vi "Main.vi"(11 "Module Admin":refnum<class "Delacor_lib_QMH_Module Admin.lvclass">) -> ()   [LabVIEW 2018, in "Storage.lvlib"]
doc: "This template is based off of the Queued Message Handler design pattern and the Queued Message Handler project template that ships with LabVIEW.\n\nThe main difference is that the queue is private to this module and communication between modules is performed via Broadcast and Request events.\n\nRequest events are wrapped in public API methods and are handled in the Event Handling Loop (EHL) of this VI. Any module can register for Broadcast events sent by this module. The EHL generates messages based on user interface actions.\n\nThe Message Handling Loop (MHL) processes messages generated by the EHL, or by other messages. The messages are string values, so new messages can be added easily to the Message Cases case structure in the MHL. Each message cluster can also provide an optional value for Message Data, which is a variant that can be converted to whatever message-specific data is required.\n_____\nBased on DQMH Project Template 6.1.0.94."
uses:
  Storage.lvlib
  <vilib>/Delacor/Delacor QMH/Libraries/Module Admin_class/Delacor_lib_QMH_Module Admin.lvclass
  Module Data--cluster.ctl
  <vilib>/drjdpowell/SQLite Library/SQL Connection/Connection.lvclass
  <vilib>/Delacor/Delacor QMH/Libraries/Message Queue_class/Delacor_lib_QMH_Message Queue.lvclass/Delacor_lib_QMH_Message Queue.ctl
  Stop Argument--cluster.ctl
  <vilib>/Delacor/Delacor QMH/Libraries/Module Admin_class/Delacor_lib_QMH_Module Admin.lvclass/Delacor_lib_QMH_Module Admin.ctl
  Get TDMS Ref Argument--cluster.ctl
  Get TDMS Ref (Reply Payload)--cluster.ctl
  <vilib>/Utility/miscctls.llb/LVPointTypeDef.ctl
  <vilib>/Utility/sysdir.llb/System Directory Type.ctl
  <vilib>/Delacor/Delacor QMH/Libraries/Message Queue_class/Delacor_lib_QMH_Enqueue Message (Single).vi
  <vilib>/Delacor/Delacor QMH/Libraries/Module Admin_class/Delacor_lib_QMH_Get External Launch.vi
  <vilib>/Delacor/Delacor QMH/Libraries/Message Queue_class/Delacor_lib_QMH_Enqueue Message (Array).vi
  <vilib>/Utility/error.llb/Error Cluster From Error Code.vi
  <vilib>/ErrorRing/Error Ring.xnode
  <vilib>/Delacor/Delacor QMH/Libraries/Message Queue_class/Delacor_lib_QMH_Message Queue.lvclass
panel:
  out "error out":errorcluster
  out "Status":string
  in  "Simulate MHL Error":bool
  in  "Simulate EHL Error":bool
  # "Other QMH Modules communicate with this Module via its Public API (wrappers for its Request Events).\n\nThis Module communicates with other Modules via its Broadcast Events.\nAny module that wants to get these messages, just registers for this module's Broadcast events."
  # "This template is for the Delacor Modified Queued Message Handler design pattern.\n\nSee the block diagram for more information on how to use this template."
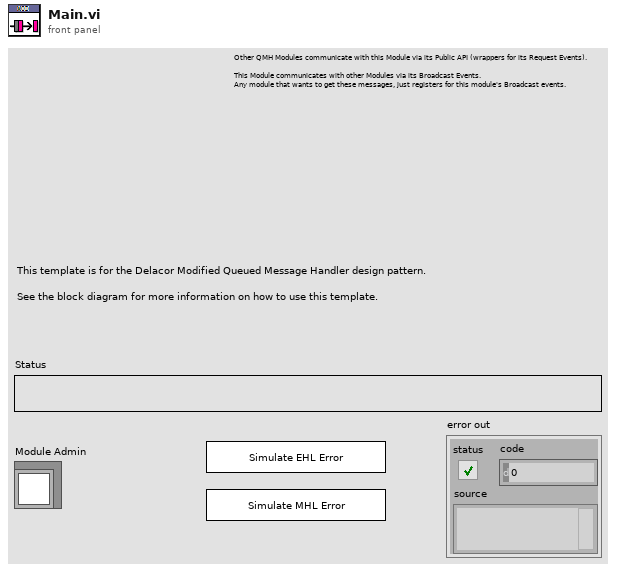
[diagram p1: front panel]
types:
  T1 = typedef "Storage.lvlib/Module Data--cluster.ctl" = cluster{"Status":string, "Data Path":path, "TDMS原":refnum<k34>[], "TDMS实":refnum<k34>[], "DB Con":refnum<class "Connection.lvclass">}
  T2 = typedef "Storage.lvlib/Request Events--cluster.ctl" = cluster{"Stop Module":refnum<user-event>, "Show Panel":refnum<user-event>, "Hide Panel":refnum<user-event>, "Get Module Execution Status":refnum<user-event>, "Show Diagram":refnum<user-event>, "Wakeup or Sleep HL":refnum<user-event>, "Get TDMS Ref":refnum<user-event>}
  T3 = enum32{"invalid lock state", "Not Locked", "Locked (No Password)", "Password-protected"}
  T4 = typedef "Storage.lvlib/Stop Argument--cluster.ctl" = cluster{"Origin":string, "Exit via Stop Module Req?":bool, "Wait for Module to stop?":bool}
  T5 = typedef "Storage.lvlib/Get TDMS Ref Argument--cluster.ctl" = cluster{"TDMS ID":i32, "Wait Notifier":refnum<notifier>, "wait for reply":bool}
  T6 = typedef "LVPointTypeDef.ctl" = cluster{"Horizontal":i16, "Vertical":i16}
  T7 = enum32{"Invalid", "Standard", "Closed", "Hidden", "Minimized", "Maximized"}
  T8 = enum16{"open", "open or create", "create or replace", "create", "open (read-only)"}
  T9 = typedef "Storage.lvlib/Get TDMS Ref (Reply Payload)--cluster.ctl" = cluster{"TDMS":refnum<k34>, "error":errorcluster}
  T10 = typedef "System Directory Type.ctl" = i32
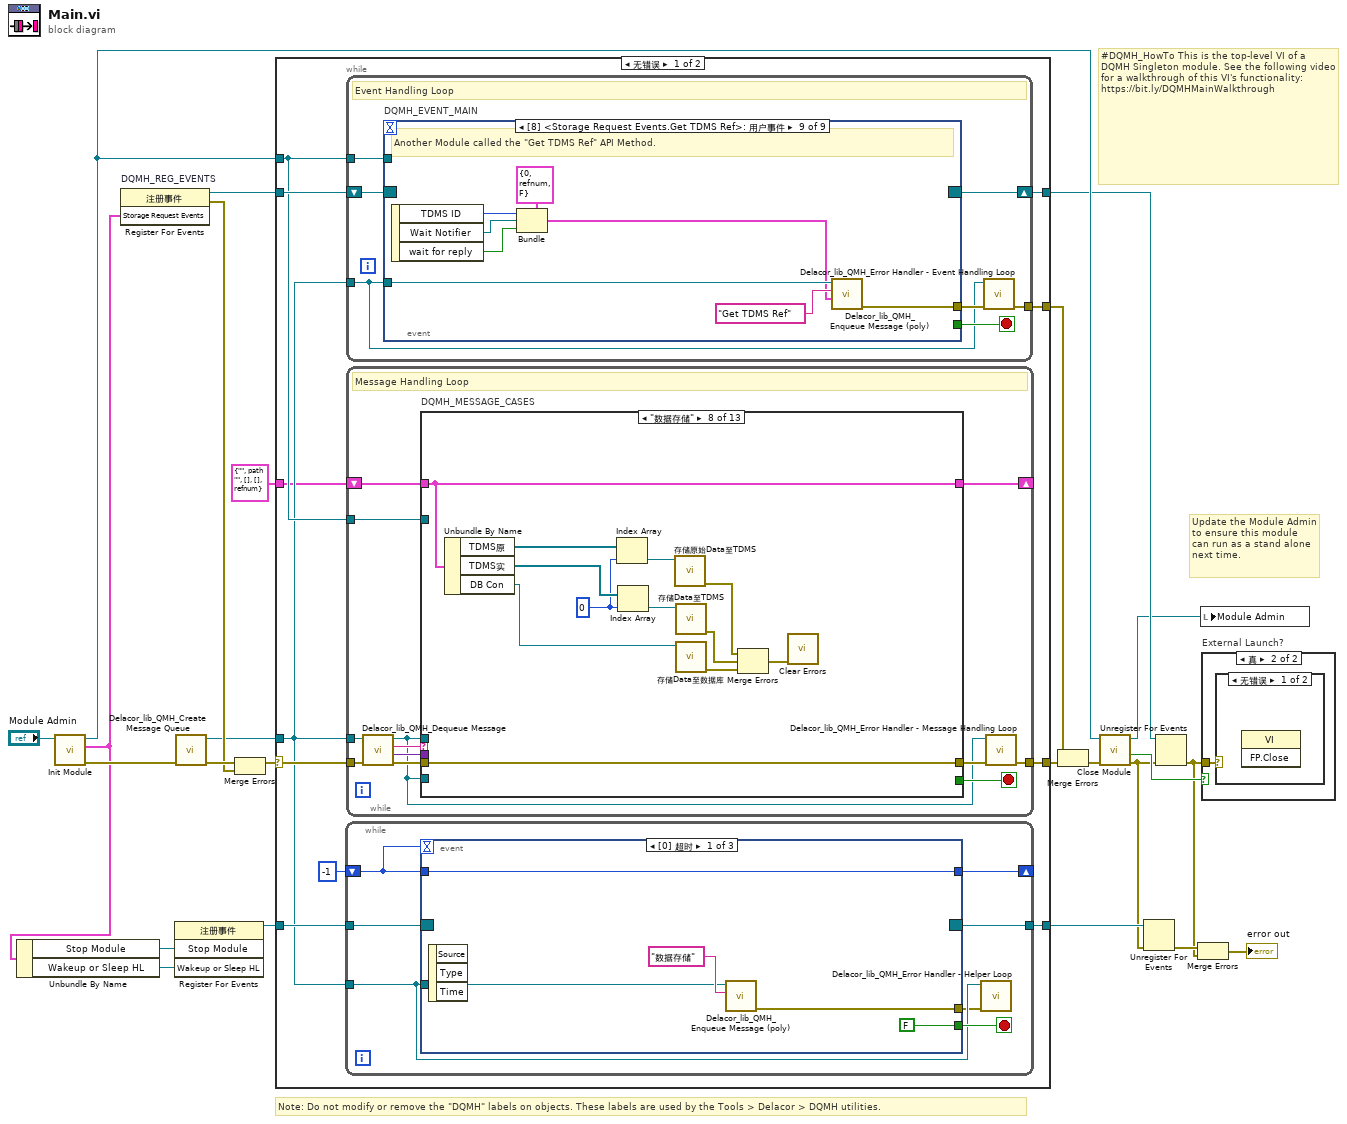
[diagram p0: block diagram]
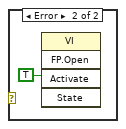
[diagram p3: hidden frame]
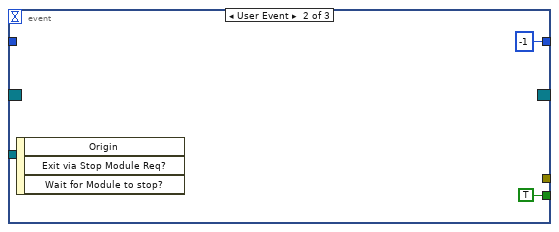
[diagram p4: hidden frame]
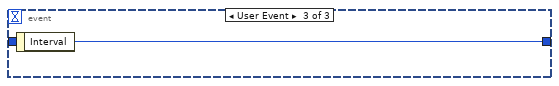
[diagram p5: hidden frame]
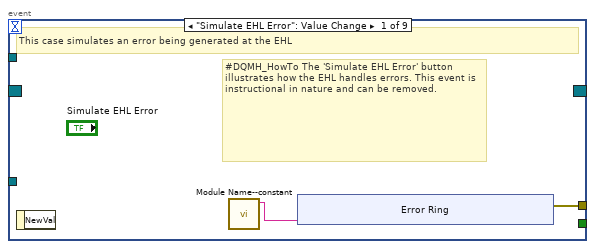
[diagram p6: hidden frame]
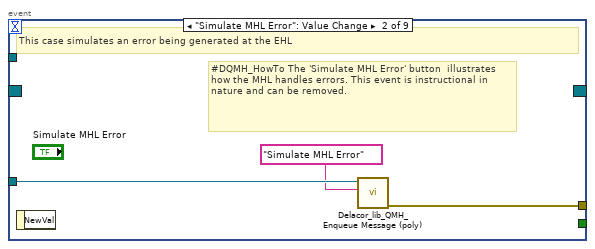
[diagram p7: hidden frame]
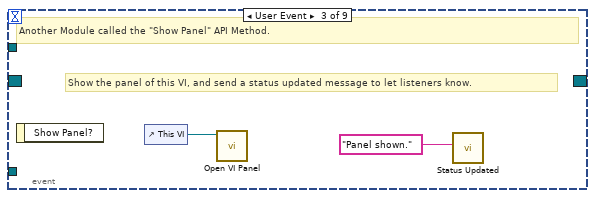
[diagram p8: hidden frame]
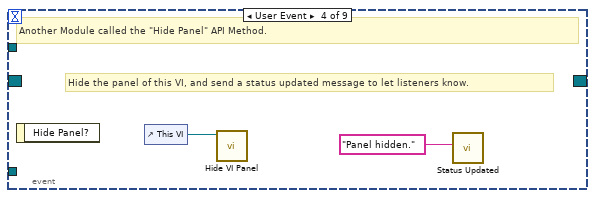
[diagram p9: hidden frame]
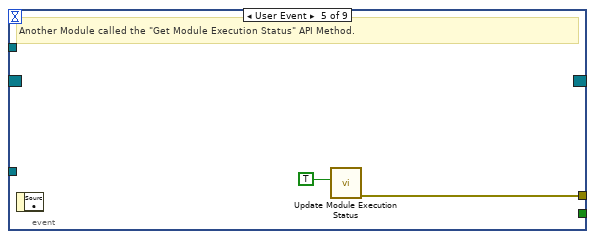
[diagram p10: hidden frame]
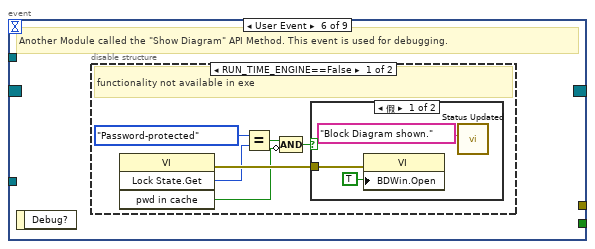
[diagram p11: hidden frame]
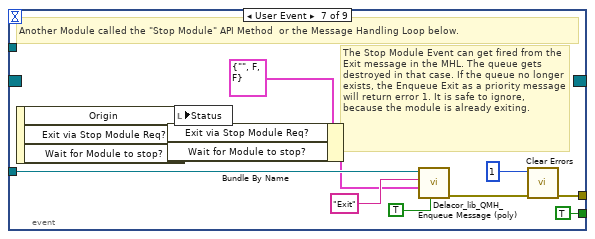
[diagram p14: hidden frame]
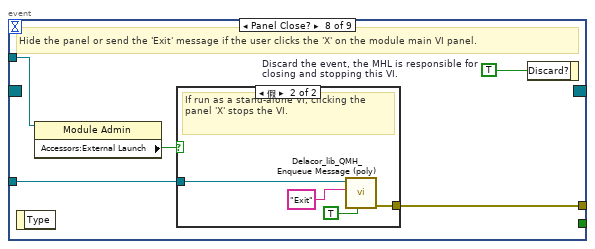
[diagram p15: hidden frame]
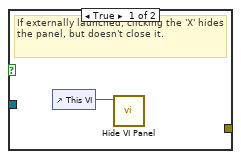
[diagram p16: hidden frame]
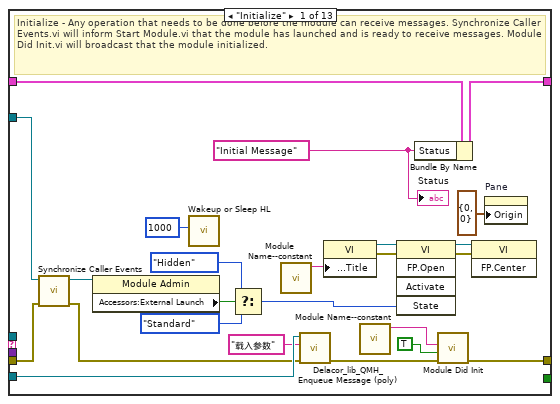
[diagram p17: hidden frame]
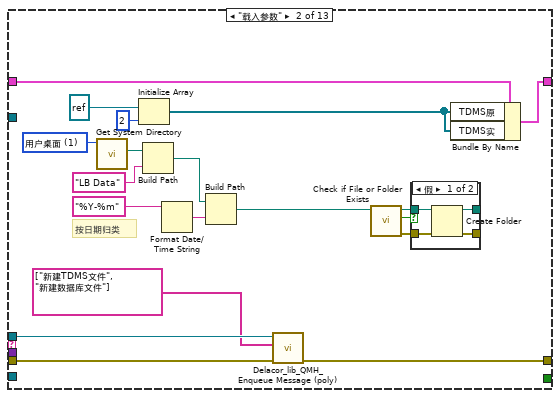
[diagram p18: hidden frame]
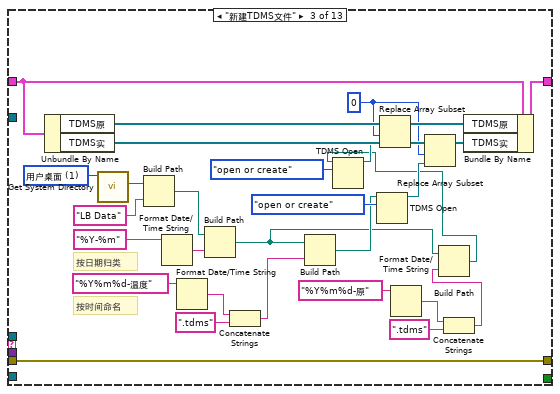
[diagram p20: hidden frame]
diagram:
  # "#DQMH_HowTo This is the top-level VI of a DQMH Singleton module. See the following video for a walkthrough of this VI's functionality: https://bit.ly/DQMHMainWalkthrough"
  # "Note: Do not modify or remove the \"DQMH\" labels on objects. These labels are used by the Tools > Delacor > DQMH utilities."
  # "Update the Module Admin to ensure this module can run as a stand alone next time."
  n1 = call "Init Module.vi"("Singleton Module Admin in"="Module Admin") -> ("error out"=w23:errorcluster, "Storage Request Events"=w7:T2, "Singleton Module Admin out"=w17:refnum<class "Delacor_lib_QMH_Module Admin.lvclass">)  [unwired: 8 in]
  n2 = Unbundle By Name ("按名称解除捆绑")(w7) -> ("Stop Module"=w10:refnum<user-event>, "Wakeup or Sleep HL"=w9:refnum<user-event>)
  n3 = register-events "DQMH_REG_EVENTS"(w7) -> (reference out=w15:refnum<event-registration>, error out=w18:errorcluster)  [unwired: 2 in]
  n4 = register-events ("注册事件")(w10, w9) -> (reference out=w8:refnum<event-registration>)  [unwired: 2 in, 1 out]
  n5 = call <vilib>:"Delacor_lib_QMH_Create Message Queue.vi"("error in"=w23) -> ("error out"=w20:errorcluster, "Message Queue"=w14:refnum<class "Delacor_lib_QMH_Message Queue.lvclass">)  [unwired: 9 in]
  n6 = Merge Errors(w20, w18) -> (w19:errorcluster)
  n7 = case shown="无错误" w19 {
    selector: w19 -> [w33 w313]
    tunnel: [w35 w312] -> w24
    tunnel: [w32 w318] -> w16
    tunnel: w15 -> [w31 w318]
    tunnel: w14 -> [w27 w311]
    tunnel: [w34 _] -> w22
    tunnel: w17 -> [w30 w314]
    tunnel: w8 -> [w28 w310]
    tunnel: [w26 w310] -> w5
    tunnel: T1 {"Status"="", "Data Path"=path "", "TDMS原"=[], "TDMS实"=[], "DB Con"=refnum} ("Data Cluster") -> [w25 _]
    frame No Error {
      n8 = while {
        shift-right: [w41] -> _
        shift-left: -1 ("Interval") -> [w42]
        tunnel: w28 -> [w39]
        tunnel: [w38] -> w26
        tunnel: w27 -> [w37]
        stop <- w40 stop-if-true
        n9 = event "事件结构" shown="[0] 超时" {
          selector: w39 -> [_ _ _]
          dyn-events: [_ _ _] -> w38
          timeout: w42 -> [_ _ _]
          tunnel: w42 -> [w43 _ _]
          tunnel: [w43 -1 w50] -> w41
          tunnel: [FALSE TRUE _] -> w40
          tunnel: w37 -> [w45 _ _]
          tunnel: [w44 _ _] -> w36
          event Timeout {
            n10 = event-data() -> ()  [unwired: 1 in, 3 out]
            n11 = call-poly <vilib>:"Delacor_lib_QMH_Enqueue Message (poly).vi"("Message"="数据存储", "Message Queue in"=w45) -> ("error out"=w44:errorcluster)  [unwired: 8 in, 1 out]
          }
          event User Event {
            n12 = event-data() -> ()  [unwired: 1 in, 3 out]
          }
          event User Event {
            n13 = event-data() -> ("Interval"=w50:i32)  [unwired: 1 in]
          }
        }
        n14 = call-dynamic "Delacor_lib_QMH_Error Handler - Helper Loop.vi"("error in"=w36, "Message Queue in"=w37) -> ()  [unwired: 8 in, 2 out]
      }
      n15 = while {
        tunnel: w27 -> [w51]
        shift-right: [w54] -> w32
        shift-left: w31 -> [w55]
        tunnel: [w56] -> w34
        tunnel: w30 -> [w52]
        stop <- w53 stop-if-true
        # "Event Handling Loop"
        n16 = event "DQMH_EVENT_MAIN" shown="[8] <Storage Request Events.Get TDMS Ref>: 用户事件" {
          selector: w55 -> [_ _ _ _ _ _ _ _ _]
          dyn-events: [_ _ _ _ _ _ _ _ _] -> w54
          timeout: _ -> [_ _ _ _ _ _ _ _ _]
          tunnel: [_ _ _ _ _ _ TRUE ("Discard?") _ _] -> w53
          tunnel: w51 -> [_ w68 _ _ _ _ w92 w99 w114]
          tunnel: [w59 w69 _ _ w75 _ w95 w101 w107] -> w57
          tunnel: w52 -> [_ _ _ _ _ _ _ w98 _]
          event "Simulate EHL Error": Value Change {
            # "#DQMH_HowTo The 'Simulate EHL Error' button  illustrates how the EHL handles errors. This event is instructional in nature and can be removed."
            # "This case simulates an error being generated at the EHL"
            n17 = event-data() -> ()  [unwired: 1 in, 1 out]
            n18 = call "Module Name--constant.vi"() -> ("Module Name"=w58:string)  [unwired: 11 in]
            n19 = xnode "Error Ring"("参数 0"=w58) -> ("错误输出"=w59:errorcluster)
          }
          event "Simulate MHL Error": Value Change {
            # "#DQMH_HowTo The 'Simulate MHL Error' button  illustrates how the MHL handles errors. This event is instructional in nature and can be removed."
            # "This case simulates an error being generated at the EHL"
            n20 = event-data() -> ()  [unwired: 1 in, 1 out]
            n21 = call-poly <vilib>:"Delacor_lib_QMH_Enqueue Message (poly).vi"("Message"="Simulate MHL Error", "Message Queue in"=w68) -> ("error out"=w69:errorcluster)  [unwired: 8 in, 1 out]
          }
          event User Event {
            # "Show the panel of this VI, and send a status updated message to let listeners know."
            # "Another Module called the \"Show Panel\" API Method."
            n22 = event-data() -> ()  [unwired: 1 in, 1 out]
            n23 = control-ref of="This VI"() -> (w71:refnum<vi>)
            n24 = call "Open VI Panel.vi"("VI"=w71) -> ()  [unwired: 10 in, 1 out]
            n25 = call "Status Updated.vi"("Status"="Panel shown." ("format string")) -> ()  [unwired: 10 in, 1 out]
          }
          event User Event {
            # "Hide the panel of this VI, and send a status updated message to let listeners know."
            # "Another Module called the \"Hide Panel\" API Method."
            n26 = event-data() -> ()  [unwired: 1 in, 1 out]
            n27 = control-ref of="This VI"() -> (w73:refnum<vi>)
            n28 = call "Hide VI Panel.vi"("VI"=w73) -> ()  [unwired: 10 in, 1 out]
            n29 = call "Status Updated.vi"("Status"="Panel hidden." ("format string")) -> ()  [unwired: 10 in, 1 out]
          }
          event User Event {
            # "Another Module called the \"Get Module Execution Status\" API Method."
            n30 = event-data() -> ()  [unwired: 1 in, 1 out]
            n31 = call "Update Module Execution Status.vi"("Running?"=TRUE) -> ("error out"=w75:errorcluster)  [unwired: 10 in]
          }
          event User Event {
            # "Another Module called the \"Show Diagram\" API Method. This event is used for debugging."
            n32 = event-data() -> ()  [unwired: 1 in, 1 out]
            n33 = disable-structure shown="RUN_TIME_ENGINE==False" {
              frame condition #0 (active) {
                # "functionality not available in exe"
                n34 = invoke class="VI" method="Lock State.Get"() -> (error out=w81:errorcluster, "Get Lock State"=w80:T3, "pwd in cache"=w77:bool)  [unwired: 4 in, 1 out]
                n35 = Equal?(x=T3."Password-protected", y=w80) -> (x = y?=w78:bool)
                n36 = Compound Arithmetic op=AND(w78, invert w77) -> (w76:bool)
                n37 = case "条件结构" shown="假" w76 {
                  tunnel: w81 -> [w84 _]
                  frame False {
                    n38 = property class="VI"(error in=w84, "BDWin.Open"=TRUE ("Block Diagram Window:Open")) -> ()  [unwired: 1 in, 2 out]
                    n39 = call "Status Updated.vi"("Status"="Block Diagram shown." ("format string")) -> ()  [unwired: 10 in, 1 out]
                  }
                  frame True {
                    # "Password-protected VI, and the password is not in the cache. Do not show the diagram."
                  }
                }
              }
              frame condition #1 {
              }
            }
          }
          event User Event {
            # "The Stop Module Event can get fired from the Exit message in the MHL. The queue gets destroyed in that case. If the queue no longer exists, the Enqueue Exit as a priority message will return error 1. It is safe to ignore, because the module is already exiting."
            # "Another Module called the \"Stop Module\" API Method  or the Message Handling Loop below."
            n40 = event-data() -> ("Origin"=w91:string, "Exit via Stop Module Req?"=w87:bool, "Wait for Module to stop?"=w86:bool)  [unwired: 1 in]
            n41 = Bundle By Name(cluster=T4 {"Origin"="", "Exit via Stop Module Req?"=FALSE, "Wait for Module to stop?"=FALSE} ("Stop Argument"), "Exit via Stop Module Req?"=w87, "Wait for Module to stop?"=w86) -> (w85:T4)
            n42 = local write "Status"(w91) -> ()
            n43 = call-poly <vilib>:"Delacor_lib_QMH_Enqueue Message (poly).vi"("Priority Message? (F)"=TRUE, "Message Data"=w85, "Message"="Exit", "Message Queue in"=w92) -> ("error out"=w96:errorcluster)  [unwired: 6 in, 1 out]
            n44 = call <vilib>:"Clear Errors.vi"("error in (no error)"=w96, "specific error code to clear (0: all)"=1) -> ("error out"=w95:errorcluster)  [unwired: 4 in, 1 out]
          }
          event Panel Close? {
            w100 = TRUE  # Discard the event, the MHL is responsible for closing and stopping this VI.
            # "Hide the panel or send the 'Exit' message if the user clicks the 'X' on the module main VI panel."
            n45 = event-data() -> ()  [unwired: 1 in, 1 out]
            n46 = property class="Module Admin"(reference=w98) -> ("Accessors:External Launch"=w97:bool)  [unwired: 1 in, 2 out]
            n47 = case "条件结构" shown="假" w97 {
              tunnel: w99 -> [_ w105]
              tunnel: [_ w106] -> w101
              frame True {
                # "If externally launched, clicking the 'X' hides the panel, but doesn't close it."
                n48 = control-ref of="This VI"() -> (w102:refnum<vi>)
                n49 = call "Hide VI Panel.vi"("VI"=w102) -> ()  [unwired: 10 in, 1 out]
              }
              frame False {
                # "If run as a stand-alone VI, clicking the panel 'X' stops the VI."
                n50 = call-poly <vilib>:"Delacor_lib_QMH_Enqueue Message (poly).vi"("Priority Message? (F)"=TRUE, "Message"="Exit", "Message Queue in"=w105) -> ("error out"=w106:errorcluster)  [unwired: 7 in, 1 out]
              }
            }
            n51 = event-data("Discard?"=w100) -> ()  [unwired: 1 in, 1 out]
          }
          event User Event {
            # "Another Module called the \"Get TDMS Ref\" API Method."
            n52 = event-data() -> ("TDMS ID"=w110:i32, "Wait Notifier"=w109:refnum<notifier>, "wait for reply"=w108:bool)  [unwired: 1 in]
            n53 = Bundle(cluster=T5 {"TDMS ID"=0, "Wait Notifier"=refnum, "wait for reply"=FALSE} ("Get TDMS Ref Argument"), "TDMS ID"=w110, "Wait Notifier"=w109, "wait for reply"=w108) -> (w111:T5)
            n54 = call-poly <vilib>:"Delacor_lib_QMH_Enqueue Message (poly).vi"("Message Data"=w111, "Message"="Get TDMS Ref", "Message Queue in"=w114) -> ("error out"=w107:errorcluster)  [unwired: 7 in, 1 out]
          }
        }
        n55 = call-dynamic "Delacor_lib_QMH_Error Handler - Event Handling Loop.vi"("error in"=w57, "Message Queue in"=w51) -> ("dup error in"=w56:errorcluster)  [unwired: 8 in, 1 out]
      }
      n56 = while {
        tunnel: w27 -> [w117]
        shift-right: [w121] -> _
        shift-left: w25 -> [w122]
        tunnel: w33 -> [w125]
        tunnel: [w123] -> w35
        tunnel: w30 -> [w116]
        stop <- w120 stop-if-true
        # "Message Handling Loop"
        n57 = call-dynamic "Delacor_lib_QMH_Dequeue Message.vi"("error in"=w125, "Message Queue in"=w117) -> ("error out"=w124:errorcluster, "Message Data"=w118:variant, "Message"=w119:string, "Message Queue out"=w115:refnum<class "Delacor_lib_QMH_Message Queue.lvclass">)  [unwired: 6 in]
        n58 = case "DQMH_MESSAGE_CASES" shown="\"数据存储\"" w119 {
          selector: w119 -> [_ _ _ _ _ _ _ _ _ _ _ _ w297]
          tunnel: w115 -> [_ w159 _ _ _ _ _ _ _ _ w258 w283 _]
          tunnel: w124 -> [w148 w158 w204 w208 w210 w224 w229 w239 w243 w248 w265 w289 w299]
          tunnel: [w147 w157 w204 w208 w210 w215 w228 w239 w243 w247 w261 w286 w300] -> w126
          tunnel: w122 -> [w138 w167 w189 w207 w209 w214 w227 w241 w242 w245 w260 w275 w298]
          tunnel: [w137 w166 w191 w206 w209 w214 w227 w241 w242 w245 w260 w275 w298] -> w121
          tunnel: [_ _ _ _ _ _ _ _ _ _ _ w282 _] -> w120
          tunnel: w118 -> [_ _ _ _ _ w222 _ _ _ _ w259 w281 _]
          tunnel: w116 -> [w139 _ _ _ _ _ _ _ _ _ w257 w276 _]
          tunnel: w115 -> [w130 _ _ _ _ _ _ _ _ _ _ _ _]
          frame "Initialize" {
            w133 = "Initial Message" ("Initial Message")
            # "Initialize - Any operation that needs to be done before the module can receive messages. Synchronize Caller Events.vi will inform Start Module.vi that the module has launched and is ready to receive messages. Module Did Init.vi will broadcast that the module initialized."
            n59 = call "Synchronize Caller Events.vi"("error in (no error)"=w148, "Singleton Module Admin in"=w139) -> ("error out"=w129:errorcluster, "Singleton Module Admin out"=w134:refnum<class "Delacor_lib_QMH_Module Admin.lvclass">)  [unwired: 8 in]
            n60 = property class="Module Admin"(reference=w134) -> ("Accessors:External Launch"=w143:bool)  [unwired: 1 in, 2 out]
            n61 = call "Wakeup or Sleep HL.vi"("Interval"=1000) -> ()  [unwired: 10 in, 1 out]
            n62 = Select(t=T7."Hidden" ("State"), s=w143, f=T7."Standard" ("State")) -> (s? t:f=w140:T7)
            n63 = call "Module Name--constant.vi"() -> ("Module Name"=w146:string)  [unwired: 11 in]
            n64 = call-poly <vilib>:"Delacor_lib_QMH_Enqueue Message (poly).vi"("error in"=w129, "Message"="载入参数", "Message Queue in"=w130) -> ("error out"=w128:errorcluster)  [unwired: 7 in, 1 out]
            n65 = property class="VI"("Front Panel.Title"=w146) -> (reference out=w145:refnum<vi>, error out=w150:errorcluster)  [unwired: 2 in]
            n66 = call "Module Name--constant.vi"() -> ("Module Name"=w135:string)  [unwired: 11 in]
            n67 = invoke class="VI" method="FP.Open"(reference=w145, error in=w150, "State"=w140) -> (reference out=w144:refnum<vi>, error out=w149:errorcluster)  [unwired: 2 in, 3 out]
            n68 = Bundle By Name(cluster=w138, "Status"=w133) -> (w137:T1)
            n69 = call "Module Did Init.vi"("error in (no error)"=w128, "Initialized?"=TRUE, "Origin"=w135) -> ("error out"=w147:errorcluster)  [unwired: 8 in]
            n70 = invoke class="VI" method="FP.Center"(reference=w144, error in=w149) -> ()  [unwired: 1 in, 3 out]
            n71 = property on="Pane" class="Pane"("Origin"=T6 {"Horizontal"=0, "Vertical"=0}) -> ()  [unwired: 2 in, 2 out]
            "Status" <- w133
          }
          frame "载入参数" {
            w165 = T10 1 items=["用户目录"=0, "用户桌面"=1, "用户文档"=2, "用户应用程序数据"=3, "用户设置"=4, "用户临时目录"=5, "公共文档"=6, "公共应用程序数据"=7, "公共设置"=8, "公共缓存"=13, "系统核心库"=9, "系统安装库"=10, "应用程序文件"=11, "启动盘根目录"=12] ("system directory type")
            # "按日期归类"
            n72 = call <vilib>:"Get System Directory.vi"("system directory type"=w165) -> ("system directory"=w164:path)  [unwired: 10 in]
            n73 = Initialize Array(refnum<k34> refnum ("TDMS"), 2 ("维数大小")) -> (w151:refnum<k34>[])
            n74 = Build Path(base path=w164, name or relative path="LB Data" ("名称或相对路径")) -> (appended path=w160:path)
            n75 = Format Date/Time String(time format string (%c)="%Y-%m" ("时间格式字符串(%c)")) -> (date/time string=w161:string)  [unwired: 2 in]
            n76 = Build Path(base path=w160, name or relative path=w161) -> (appended path=w152:path)
            n77 = call-poly <vilib>:"Delacor_lib_QMH_Enqueue Message (poly).vi"("error in"=w158, "Message Array"=string[] ["新建TDMS文件", "新建数据库文件"] ("Message"), "Message Queue in"=w159) -> ("error out"=w157:errorcluster)  [unwired: 7 in, 1 out]
            n78 = call <vilib>:"Check if File or Folder Exists.vi"("path"=w152) -> ("error out"=w154:errorcluster, "file or folder exists?"=w155:bool, "dup path"=w153:path)  [unwired: 8 in]
            n79 = case shown="假" w155 {
              tunnel: w153 -> [w173 w174]
              tunnel: w154 -> [w172 w175]
              tunnel: [w171 w175] -> _
              tunnel: [w170 w174] -> _
              frame False {
                n80 = Create Folder(path (use dialog)=w173, error in=w172) -> (created path=w170:path, error out=w171:errorcluster)  [unwired: 1 in, 1 out]
              }
              frame True {
              }
            }
            n81 = Bundle By Name(cluster=w167, "TDMS原"=w151, "TDMS实"=w151) -> (w166:T1)
          }
          frame "新建TDMS文件" {
            w184 = 0 ("索引")
            w203 = T10 1 items=["用户目录"=0, "用户桌面"=1, "用户文档"=2, "用户应用程序数据"=3, "用户设置"=4, "用户临时目录"=5, "公共文档"=6, "公共应用程序数据"=7, "公共设置"=8, "公共缓存"=13, "系统核心库"=9, "系统安装库"=10, "应用程序文件"=11, "启动盘根目录"=12] ("system directory type")
            # "按时间命名"
            # "按日期归类"
            n82 = Unbundle By Name(w189) -> ("TDMS原"=w186:refnum<k34>[], "TDMS实"=w188:refnum<k34>[])
            n83 = call <vilib>:"Get System Directory.vi"("system directory type"=w203) -> ("system directory"=w202:path)  [unwired: 10 in]
            n84 = Build Path(base path=w202, name or relative path="LB Data" ("名称或相对路径")) -> (appended path=w198:path)
            n85 = Format Date/Time String(time format string (%c)="%Y-%m" ("时间格式字符串(%c)")) -> (date/time string=w199:string)  [unwired: 2 in]
            n86 = Format Date/Time String(time format string (%c)="%Y%m%d-温度" ("时间格式字符串(%c)")) -> (date/time string=w196:string)  [unwired: 2 in]
            n87 = Build Path(base path=w198, name or relative path=w199) -> (appended path=w178:path)
            n88 = Concatenate Strings(w196, ".tdms" ("字符串")) -> (w194:string)
            n89 = Build Path(base path=w178, name or relative path=w194) -> (appended path=w192:path)
            n90 = TDMS Open(10:T8."open or create" ("操作(0:open)"), 11:w192) -> (3:w187:refnum<k34>)  [unwired: 5 in, 1 out]
            n91 = Format Date/Time String(time format string (%c)="%Y%m%d-原" ("时间格式字符串(%c)")) -> (date/time string=w180:string)  [unwired: 2 in]
            n92 = Replace Array Subset(array=w188, new element=w187, index=w184) -> (w190:refnum<k34>[])
            n93 = Concatenate Strings(w180, ".tdms" ("字符串")) -> (w177:string)
            n94 = Build Path(base path=w178, name or relative path=w177) -> (appended path=w176:path)
            n95 = TDMS Open(10:T8."open or create" ("操作(0:open)"), 11:w176) -> (3:w183:refnum<k34>)  [unwired: 5 in, 1 out]
            n96 = Replace Array Subset(array=w186, new element=w183, index=w184) -> (w185:refnum<k34>[])
            n97 = Bundle By Name(cluster=w189, "TDMS原"=w185, "TDMS实"=w190) -> (w191:T1)
          }
          frame "新建数据库文件" {
            n98 = call "DB_创建Temperature表.vi"() -> ("SQLite Connection"=w205:refnum<class "Connection.lvclass">)  [unwired: 10 in, 1 out]
            n99 = Bundle By Name(cluster=w207, "DB Con"=w205) -> (w206:T1)
          }
          frame "---Module Specific---" {
            # "Separator -- The following cases handle messages specific to this Module."
          }
          frame "Get TDMS Ref" {
            n100 = Variant To Data(error in=w224, type=T5 {"TDMS ID"=0, "Wait Notifier"=refnum, "wait for reply"=FALSE} ("Get TDMS Ref Argument"), Variant=w222) -> (data=w220:T5, error out=w223:errorcluster)
            n101 = Unbundle By Name(w214) -> ("TDMS实"=w213:refnum<k34>[])
            n102 = Unbundle By Name(w220) -> ("TDMS ID"=w212:i32, "Wait Notifier"=w219:refnum<notifier>, "wait for reply"=w218:bool)
            n103 = Index Array(array=w213, index=w212) -> (element=w211:refnum<k34>)
            n104 = Merge Errors(w223) -> (w215:errorcluster)
            n105 = Bundle By Name(cluster=T9 {"TDMS"=refnum, "error"={"status"=FALSE, "code"=0, "source"=""}} ("Get TDMS Ref (Reply Payload)"), "TDMS"=w211) -> (w217:T9)
            n106 = case shown="真" w218 {
              tunnel: w219 -> [_ w226]
              tunnel: w217 -> [_ w225]
              frame False {
              }
              frame True {
                n107 = Send Notification(notification=w225, notifier=w226) -> ()  [unwired: 1 in, 2 out]
              }
            }
          }
          frame "---Copy This Frame---" {
            # "Duplicate this frame when creating new messages.  Change this comment in the duplicated frame to describe this message."
            n108 = Merge Errors(w229) -> (w228:errorcluster)
          }
          frame "数据存储" {
            w232 = 0 ("索引")
            n109 = Unbundle By Name(w241) -> ("TDMS原"=w233:refnum<k34>[], "TDMS实"=w240:refnum<k34>[], "DB Con"=w238:refnum<class "Connection.lvclass">)
            n110 = Index Array(array=w233, index=w232) -> (element=w231:refnum<k34>)
            n111 = Index Array(array=w240, index=w232) -> (element=w237:refnum<k34>)
            n112 = call "存储原始Data至TDMS.vi"("TDMS"=w231) -> ("error out"=w230:errorcluster)  [unwired: 9 in, 1 out]
            n113 = call "存储Data至TDMS.vi"("TDMS"=w237) -> ("error out"=w235:errorcluster)  [unwired: 9 in, 1 out]
            n114 = call "存储Data至数据库.vi"("DB Con"=w238) -> ("error out"=w236:errorcluster)  [unwired: 9 in, 1 out]
            n115 = Merge Errors(w230, w235, w236) -> (w234:errorcluster)
            n116 = call <vilib>:"Clear Errors.vi"("error in (no error)"=w234) -> ()  [unwired: 5 in, 2 out]
          }
          frame "---Exit and Error Handling---" {
            # "Separator - The following cases handle errors and exit messages."
          }
          frame "Simulate MHL Error" {
            # "#DQMH_HowTo The 'Simulate MHL Error' button  illustrates how the MHL handles errors. This event is instructional in nature and can be removed."
            # "Simulate an error occurring at the MHL"
            n117 = call "Module Name--constant.vi"() -> ("Module Name"=w244:string)  [unwired: 11 in]
            n118 = xnode "Error Ring"("参数 0"=w244) -> ("错误输出"=w246:errorcluster)
            n119 = Merge Errors(w248, w246) -> (w247:errorcluster)
          }
          frame "Error" {
            # "#CodeRecommended - If you ever change the name of this \"Error\" message, you'll need to update the name in the Check Loop Error.vi as well."
            # "#CodeRecommended - If the module is running in standalone mode (External Launch = FALSE), this code will pop up an error dialog and call the 'Exit' message if an error occurs. Add more fine-grained error handling here."
            # "Error - Check the error message data and respond accordingly. This message is sent by the \"Error Handler\" VIs at the end of each loop in this application."
            n120 = property class="Module Admin"(reference=w257) -> ("Accessors:External Launch"=w256:bool)  [unwired: 1 in, 2 out]
            n121 = Variant To Data(error in=w265, type=errorcluster {"status"=FALSE, "code"=0, "source"=""} ("error constant"), Variant=w259) -> (data=w266:errorcluster, error out=w263:errorcluster)
            n122 = call "Error Reported.vi"("Error"=w266) -> ()  [unwired: 10 in, 1 out]
            n123 = case shown="假" w256 {
              tunnel: [w271 _] -> w262
              tunnel: w258 -> [w269 _]
              tunnel: w266 -> [w270 _]
              frame False {
                # "If the module is running standalone, then pop up an error dialog and call the \"Exit\" message."
                n124 = call <vilib>:"Simple Error Handler.vi"("error in (no error)"=w270) -> ()  [unwired: 4 in, 5 out]
                n125 = call-poly <vilib>:"Delacor_lib_QMH_Enqueue Message (poly).vi"("Priority Message? (F)"=TRUE, "Message"="Exit", "Message Queue in"=w269) -> ("error out"=w271:errorcluster)  [unwired: 7 in, 1 out]
              }
              frame True {
                # "If the module was launched externally, calling the Error Reported broadcast VI is the only action performed by the \"Error\" message. The module's caller can then process the error appropriately."
              }
            }
            n126 = Merge Errors(w263, w262) -> (w261:errorcluster)
            n127 = local write "error out"(w261) -> ()
          }
          frame "Exit" {
            w280 = 91  # 91: not all Exit messages will have an argument
            w282 = TRUE  # Stop the VI
            # "Release the message queue reference"
            # "Exit - Exit the application."
            n128 = Variant To Data(error in=w289, type=T4 {"Origin"="", "Exit via Stop Module Req?"=FALSE, "Wait for Module to stop?"=FALSE} ("Stop Argument"), Variant=w281) -> (data=w278:T4, error out=w285:errorcluster)
            n129 = Unbundle By Name(w275) -> ("TDMS原"=w274:refnum<k34>[], "TDMS实"=w272:refnum<k34>[], "DB Con"=w273:refnum<class "Connection.lvclass">)
            n130 = call <vilib>:"Clear Errors.vi"("error in (no error)"=w285, "specific error code to clear (0: all)"=w280) -> ("error out"=w288:errorcluster)  [unwired: 4 in, 1 out]
            n131 = control-ref of="This VI"() -> (w277:refnum<vi>)
            n132 = call-dynamic "Close.vi"("SQLite Connection in"=w273) -> ()  [unwired: 10 in, 1 out]
            n133 = call-dynamic "Delacor_lib_QMH_Release Message Queue.vi"("error in"=w288, "Message Queue"=w283) -> ("error out"=w287:errorcluster)  [unwired: 9 in]
            n134 = call "Handle Exit.vi"("Stop Argument"=w278, "Admin in"=w276, "VI reference"=w277) -> ("error out"=w284:errorcluster)  [unwired: 7 in, 1 out]
            n135 = for {
              tunnel: w274 -> [w293] mode=indexing
              n136 = Not A Number/Path/Refnum?(number/path/refnum=w293) -> (NaN/Path/Refnum?=w294:bool)
              n137 = case shown="假" w294 {
                tunnel: w293 -> [w295 _]
                frame False {
                  n138 = TDMS Close(11:w295) -> ()  [unwired: 1 in, 2 out]
                }
                frame True {
                }
              }
            }
            n139 = for {
              tunnel: w272 -> [w290] mode=indexing
              n140 = Not A Number/Path/Refnum?(number/path/refnum=w290) -> (NaN/Path/Refnum?=w291:bool)
              n141 = case shown="假" w291 {
                tunnel: w290 -> [w292 _]
                frame False {
                  n142 = TDMS Close(11:w292) -> ()  [unwired: 1 in, 2 out]
                }
                frame True {
                }
              }
            }
            n143 = Merge Errors(w287, w284) -> (w286:errorcluster)
          }
          frame Default {
            # "'Default' case only runs if there is a message that isn't defined in any of the other cases.  Output a programming error."
            n144 = call "Module Name--constant.vi"() -> ("Module Name"=w296:string)  [unwired: 11 in]
            n145 = xnode "Error Ring"("参数 0"=w297, "参数 1"=w296) -> ("错误输出"=w301:errorcluster)
            n146 = Merge Errors(w299, w301) -> (w300:errorcluster)
          }
        }
        n147 = call-dynamic "Delacor_lib_QMH_Error Handler - Message Handling Loop.vi"("error in"=w126, "Message Queue in"=w115) -> ("dup error in"=w123:errorcluster)  [unwired: 8 in, 1 out]
      }
    }
    frame Error {
      # "Synchronize Caller Events.vi will inform Start Module.vi that the module has launched and will let the code calling Start Module.vi register for broadcasts and would permit the caller receive the broadcast that an error occurred at launch time."
      n148 = call-dynamic "Delacor_lib_QMH_Release Message Queue.vi"("error in"=w313, "Message Queue"=w311) -> ("error out"=w312:errorcluster)  [unwired: 9 in]
      n149 = call "Synchronize Caller Events.vi"("Singleton Module Admin in"=w314) -> ("error out"=w319:errorcluster)  [unwired: 9 in, 1 out]
      n150 = call "Module Name--constant.vi"() -> ("Module Name"=w317:string)  [unwired: 11 in]
      n151 = Format Into String(format string="An error occurred during initialization. %s is no longer running.", w317) -> (resulting string=w315:string)  [unwired: 2 in, 1 out]
      n152 = Merge Errors(w312, w319) -> (w320:errorcluster)
      n153 = call "Error Reported.vi"("Additional Information"=w315, "Error"=w320) -> ()  [unwired: 9 in, 1 out]
    }
  }
  n154 = Merge Errors(w22, w24) -> (w21:errorcluster)
  n155 = call "Close Module.vi"("error in (no error)"=w21, "Module Admin in"=w17) -> ("error out"=w2:errorcluster, "External Launch"=w11:bool, "Module Admin out"=w12:refnum<class "Delacor_lib_QMH_Module Admin.lvclass">)  [unwired: 7 in]
  n156 = Unregister For Events(event registration refnum=w5, error in=w2) -> (error out=w6:errorcluster)
  n157 = Unregister For Events(event registration refnum=w16, error in=w2) -> (error out=w4:errorcluster)
  n158 = Merge Errors(w6, w4) -> (→"error out":errorcluster)
  n159 = local write "Module Admin"(w12) -> ()
  n160 = case "External Launch?" shown="真" w11 {
    tunnel: w4 -> [_ w321]
    frame False {
    }
    frame True {
      n161 = case "条件结构" shown="无错误" w321 {
        frame No Error {
          n162 = invoke class="VI" method="FP.Close"() -> ()  [unwired: 3 in, 3 out]
        }
        frame Error {
          n163 = invoke class="VI" method="FP.Open"("Activate"=TRUE ("Activate?")) -> ()  [unwired: 4 in, 5 out]
        }
      }
    }
  }
